vi "Log.vi"(6 "Timeout":bool, 7 "ExecTime (ms)":i32, 8 "error in":errorcluster, 9 "Response":string, 10 "Command":string, 11 "VISA in":refnum<visa-resource-name>) -> (0 "error out":errorcluster, 2 "Log Line":string, 3 "VISA out":refnum<visa-resource-name>)   [LabVIEW 2016, in "Serial_G.lvlib"]
doc: "Logs to a text file @ \"User Documents\" folder from current windows user"
uses:
  Serial_G.lvlib
  <vilib>/Utility/sysdir.llb/System Directory Type.ctl
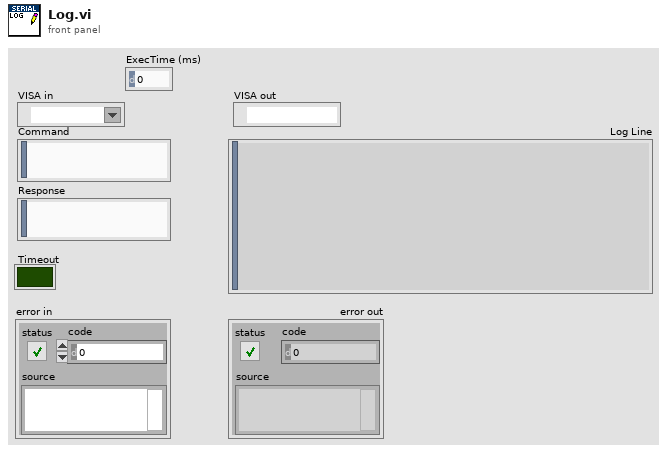
[diagram p1: front panel]
types:
  T1 = enum16{"open", "replace", "create", "open or create", "replace or create", "replace or create with confirmation"}
  T2 = typedef "System Directory Type.ctl" = i32
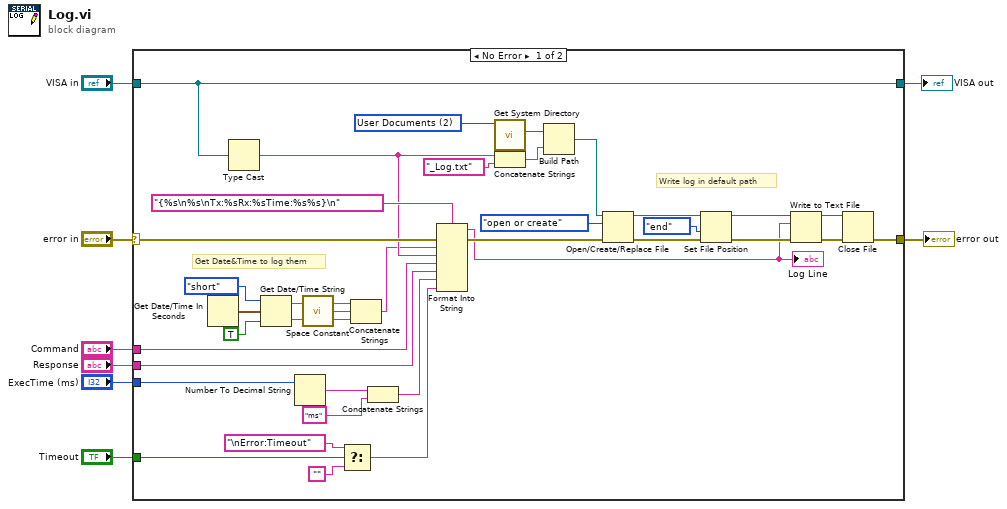
[diagram p0: block diagram]
diagram:
  n1 = case shown="No Error" "error in" {
    selector: "error in" -> [w23 w47]
    tunnel: [w43 w47] -> w8
    tunnel: "VISA in" -> [w13 w46]
    tunnel: [w13 w46] -> w5
    tunnel: "Command" -> [w12 _]
    tunnel: "Response" -> [w11 _]
    tunnel: "ExecTime (ms)" -> [w10 _]
    tunnel: "Timeout" -> [w9 _]
    frame No Error {
      w32 = T2 2 items=["User Home"=0, "User Desktop"=1, "User Documents"=2, "User Application Data"=3, "User Preferences"=4, "User Temporary"=5, "Public Documents"=6, "Public Application Data"=7, "Public Preferences"=8, "Public Cache"=13, "System Core Libraries"=9, "System Installed Libraries"=10, "Application Files"=11, "Boot Volume Root"=12] ("system directory type")
      # "Get Date&Time to log them"
      # "Write log in default path"
      n2 = Get Date/Time In Seconds() -> (seconds since 1Jan1904=w29:timestamp)
      n3 = Type Cast(x=w13) -> (*(type *) &x=w16:string)  [unwired: 1 in]
      n4 = Get Date/Time String(date format (0)=enum16{"short", "long", "abbreviated"}."short", seconds (now)=w29, want seconds? (F)=TRUE) -> (date string=w25:string, time string=w24:string)
      n5 = Number To Decimal String(number=w10) -> (decimal integer string=w22:string)  [unwired: 1 in]
      n6 = call <vilib>:"Space Constant.vi"() -> ("String"=w26:string)
      n7 = Select(t="\nError:Timeout" ("format string"), s=w9, f="" ("format string")) -> (s? t:f=w18:string)
      n8 = Concatenate Strings(w25, w26, w24) -> (w15:string)
      n9 = Concatenate Strings(w22, "ms" ("string")) -> (w17:string)
      n10 = Format Into String(format string="{%s\n%s\nTx:%sRx:%sTime:%s%s}\n", error in=w23, w15, w16, w12, w11, w17, w18) -> (resulting string=w14:string, error out=w44:errorcluster)  [unwired: 1 in]
      "Log Line" <- w14
      n11 = call <vilib>:"Get System Directory.vi"("system directory type"=w32) -> ("system directory"=w31:path)  [unwired: 10 in]
      n12 = Concatenate Strings(w16, "_Log.txt" ("name or relative path")) -> (w19:string)
      n13 = Build Path(base path=w31, name or relative path=w19) -> (appended path=w30:path)
      n14 = Open/Create/Replace File(file path (use dialog)=w30, error in=w44, operation (0:open)=T1."open or create") -> (refnum out=w38:refnum<file>, error out=w36:errorcluster)  [unwired: 3 in, 1 out]
      n15 = Set File Position(refnum=w38, from (0:start)=enum16{"start", "end", "current"}."end", error in=w36) -> (refnum out=w37:refnum<file>, error out=w35:errorcluster)  [unwired: 1 in]
      n16 = Write to Text File(file (use dialog)=w37, text=w14, error in=w35) -> (refnum out=w39:refnum<file>, error out=w40:errorcluster)  [unwired: 1 in, 1 out]
      n17 = Close File(refnum=w39, error in=w40) -> (error out=w43:errorcluster)  [unwired: 1 out]
    }
    frame Error {
    }
  }
  "error out" <- w8
  "VISA out" <- w5
